vi "CRYDataView Pane Resize Proc.vi"(8 "DataView Index":i32, 11 "VI Ref":refnum<vi>) -> ()   [LabVIEW 2013]
uses:
  CRYNew View Global.vi
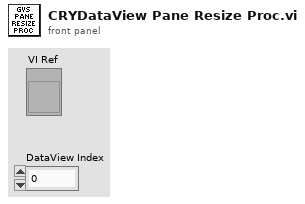
[diagram p1: front panel]
types:
  T1 = typedef "Graph Main Info Cluster.ctl" = cluster{"Selected_BarIdx":i32, "Selected_PanelIdx":i32, "Graph Main VIRef":refnum<vi>, "ToolBarClick":bool, "Spliter Ref Array":refnum<vi>[], "Panel Ref Array":refnum<vi>[], "Spliter_matrix":i32[][], "Panel_matrix":i32[][], "child_spliterIdx_matrix":i32[][], "split_pos_matrix":i32[][], "Title State":bool, "sQueueName":string, "Frame nID":i32, "Graph VIRef Array":cluster{"Graph VIRef":refnum<vi>, "Panel Idx":i32, "Frame VIRef":refnum<vi>, "Icon Ring":i32, "Graph Type":string}[], "View Type":string}
  T2 = typedef "LVRectTypeDef.ctl" = cluster{"Left":i16, "Top":i16, "Right":i16, "Bottom":i16}
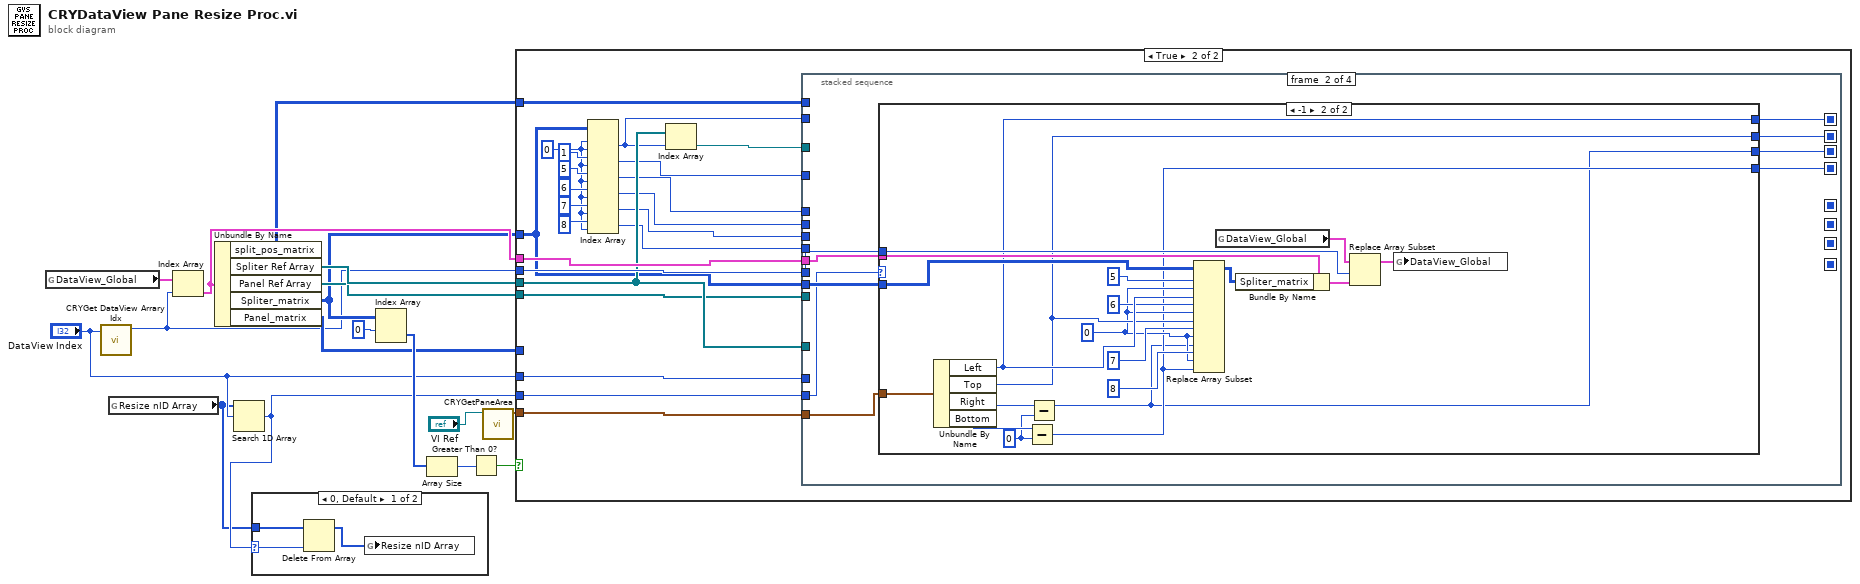
[diagram p0: block diagram]
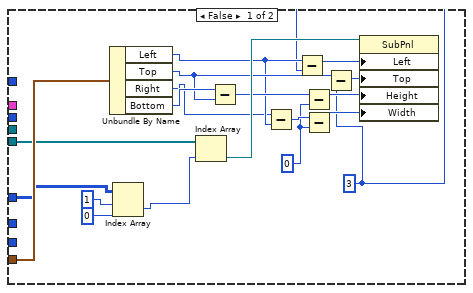
[diagram p3: hidden frame]
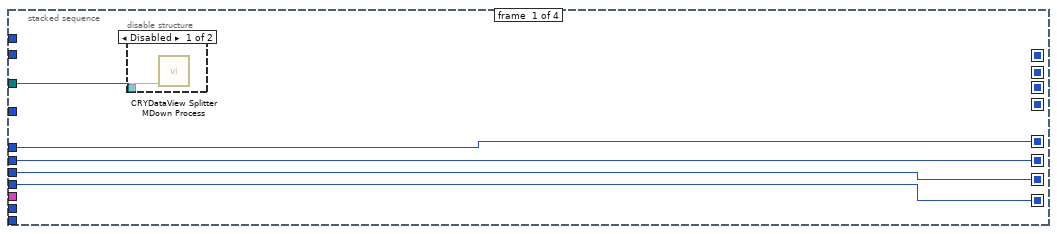
[diagram p4: hidden frame]
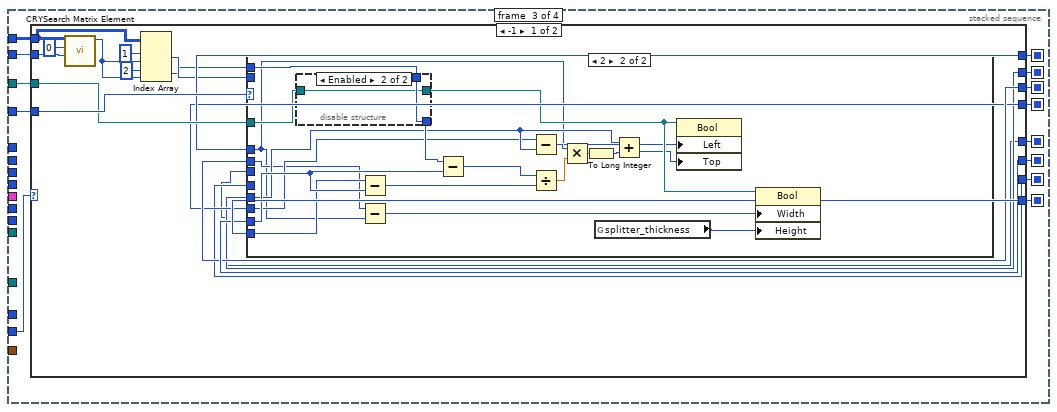
[diagram p7: hidden frame]
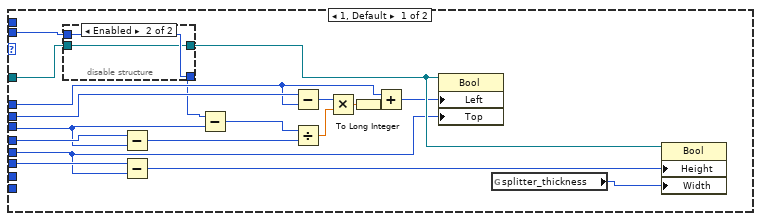
[diagram p8: hidden frame]
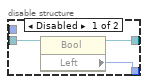
[diagram p9: hidden frame]
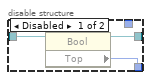
[diagram p10: hidden frame]
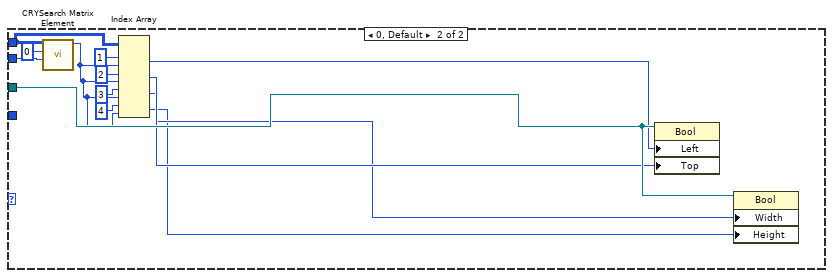
[diagram p11: hidden frame]
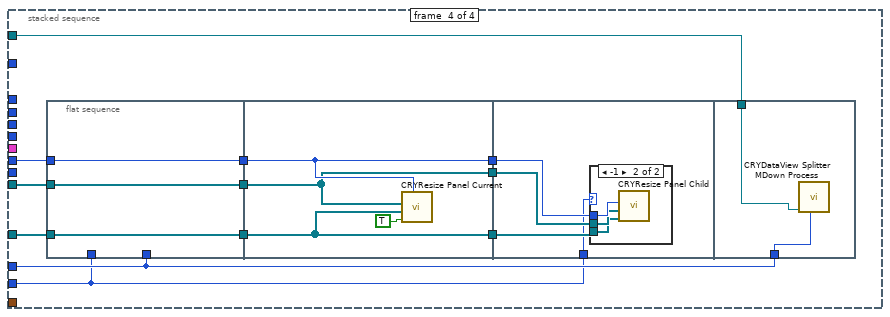
[diagram p12: hidden frame]
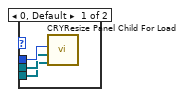
[diagram p13: hidden frame]
diagram:
  n1 = global read "CRYNew View Global.vi" "DataView_Global"() -> (w12:T1[])
  n2 = call "CRYGet DataView Arrary Idx.vi"("DataView Idx In"="DataView Index") -> ("DataView Arrary Idx out"=w5:i32)  [unwired: 10 in]
  n3 = global read "CRYNew View Global.vi" "Resize nID Array"() -> (w1:i32[])
  n4 = Index Array(array=w12, index=w5) -> (element=w13:T1)
  n5 = Unbundle By Name(w13) -> ("split_pos_matrix"=w4:i32[][], "Spliter Ref Array"=w10:refnum<vi>[], "Panel Ref Array"=w9:refnum<vi>[], "Spliter_matrix"=w6:i32[][], "Panel_matrix"=w7:i32[][])
  n6 = Search 1D Array(1D array=w1, element="DataView Index") -> (index of element=w2:i32)  [unwired: 1 in]
  n7 = case shown="0, Default" w2 {
    selector: w2 -> [w19 _]
    tunnel: w1 -> [w20 _]
    frame 0, Default {
      n8 = Delete From Array(array=w20, index=w19) -> (array with subset deleted=w18:i32[])  [unwired: 1 in, 1 out]
      n9 = global write "CRYNew View Global.vi" "Resize nID Array"(w18) -> ()
    }
    frame -1 {
    }
  }
  n10 = Index Array(array=w6, index (row)=0) -> (element=w16:i32[])  [unwired: 1 in]
  n11 = Array Size(array=w16) -> (size(s)=w15:i32)
  n12 = Greater Than 0?(x=w15) -> (x > 0?=w14:bool)
  n13 = call "CRYGetPaneArea.vi"("vi reference"="VI Ref") -> ("Content Area Rect"=w11:T2)  [unwired: 10 in]
  n14 = case shown="True" w14 {
    tunnel: w6 -> [_ w49]
    tunnel: w10 -> [_ w58]
    tunnel: w13 -> [_ w60]
    tunnel: w5 -> [_ w59]
    tunnel: w9 -> [w38 w57]
    tunnel: w11 -> [w39 w56]
    tunnel: w7 -> [w30 _]
    tunnel: "DataView Index" -> [_ w45]
    tunnel: w4 -> [_ w42]
    tunnel: w2 -> [_ w40]
    frame False {
      w21 = 3
      w24 = i16 0 ("y")
      n15 = Unbundle By Name(w39) -> ("Left"=w32:i16, "Top"=w35:i16, "Right"=w31:i16, "Bottom"=w36:i16)
      n16 = Index Array(array=w30, index (row)=1, index (col)=0) -> (element=w27:i32)
      n17 = Index Array(array=w38, index=w27) -> (element=w37:refnum<vi>)
      n18 = Subtract(x=w36, y=w35) -> (x-y=w34:i16)
      n19 = Subtract(x=w31, y=w32) -> (x-y=w33:i16)
      n20 = Subtract(x=w32, y=w21) -> (x-y=w23:i32)
      n21 = Subtract(x=w34, y=w24) -> (x-y=w25:i16)
      n22 = Subtract(x=w33, y=w24) -> (x-y=w26:i16)
      n23 = Subtract(x=w35, y=w21) -> (x-y=w22:i32)
      n24 = property class="SubPnl"(reference=w37, "Left"=w23, "Top"=w22, "Height"=w25, "Width"=w26) -> ()  [unwired: 1 in, 2 out]
    }
    frame True {
      w50 = 0 ("disabled index (col)")
      n25 = Index Array(array=w49, index (row) #1=w50, index (col) #1=w50, index (row) #2=1 ("index (row)"), index (col) #2=w50, index (row) #3=5 ("index (row)"), index (col) #3=w50, index (row) #4=6 ("index (row)"), index (col) #4=w50, index (row) #5=7 ("index (row)"), index (col) #5=w50, index (row) #6=8 ("index (row)"), index (col) #6=w50) -> (element #1=w41:i32, element #2=w48:i32, element #3=w47:i32, element #4=w46:i32, element #5=w44:i32, element #6=w43:i32)
      n26 = Index Array(array=w58, index=w41) -> (element=w61:refnum<vi>)
      n27 = stacked-sequence {
        seq-local: [w63 _ _ _] -> [_ _ w107 _]
        seq-local: [w64 _ _ _] -> [_ _ w101 _]
        seq-local: [w65 _ _ _] -> [_ _ w106 _]
        seq-local: [w66 _ _ _] -> [_ _ w100 _]
        seq-local: [_ w72 _ _] -> [_ _ w104 _]
        seq-local: [_ w71 _ _] -> [_ _ w102 _]
        seq-local: [_ w69 _ _] -> [_ _ w105 _]
        seq-local: [_ w70 _ _] -> [_ _ w103 _]
        tunnel: w61 -> [w62 _ w108 w194]
        tunnel: w60 -> [_ w76 _ _]
        tunnel: w49 -> [_ w73 _ _]
        tunnel: w59 -> [_ w75 _ w195]
        tunnel: w48 -> [_ _ w109 _]
        tunnel: w47 -> [w66 _ _ _]
        tunnel: w46 -> [w65 _ _ _]
        tunnel: w44 -> [w64 _ _ _]
        tunnel: w43 -> [w63 _ _ _]
        tunnel: w58 -> [_ _ _ w197]
        tunnel: w57 -> [_ _ _ w196]
        tunnel: w56 -> [_ w74 _ _]
        tunnel: w45 -> [_ _ _ w190]
        tunnel: w42 -> [_ _ w98 _]
        tunnel: w41 -> [_ _ w99 _]
        tunnel: w40 -> [_ w68 w97 w189]
        frame #0 {
          n28 = disable-structure shown="Disabled" {
            disable-tunnel: w62 -> [w67 _]
            frame Disabled {
              n29 = call "CRYDataView Splitter MDown Process.vi"("Selected Spliter Ref"=w67) -> ()  [unwired: 10 in, 1 out]
            }
            frame Enabled {
            }
          }
        }
        frame #1 {
          n30 = case shown="-1" w68 {
            tunnel: w76 -> [_ w96]
            tunnel: w75 -> [_ w94]
            tunnel: w74 -> [_ w91]
            tunnel: w73 -> [_ w90]
            tunnel: [_ w88] -> w72
            tunnel: [_ w86] -> w71
            tunnel: [_ w80] -> w70
            tunnel: [_ w78] -> w69
            frame 0, Default {
            }
            frame -1 {
              w77 = i16 0 ("y")
              w82 = 0 ("index (col)")
              n31 = Unbundle By Name(w91) -> ("Left"=w88:i16, "Top"=w86:i16, "Right"=w84:i16, "Bottom"=w79:i16)
              n32 = Subtract(x=w79, y=w77) -> (x-y=w80:i16)
              n33 = Subtract(x=w84, y=w77) -> (x-y=w78:i16)
              n34 = Replace Array Subset(array=w90, new element #1=w88, index (row) #1=5 ("disabled index (row)"), index (col) #1=w82, new element #2=w86, index (row) #2=6 ("disabled index (row)"), index (col) #2=w82, new element #3=w78, index (row) #3=7 ("disabled index (row)"), index (col) #3=w82, new element #4=w80, index (row) #4=8 ("disabled index (row)"), index (col) #4=w82) -> (w81:i32[][])
              n35 = global read "CRYNew View Global.vi" "DataView_Global"() -> (w92:T1[])
              n36 = Bundle By Name(cluster=w96, "Spliter_matrix"=w81) -> (w95:T1)
              n37 = Replace Array Subset(array=w92, new element=w95, index=w94) -> (w93:T1[])
              n38 = global write "CRYNew View Global.vi" "DataView_Global"(w93) -> ()
            }
          }
        }
        frame #2 {
          n39 = case shown="-1" w97 {
            tunnel: w109 -> [w127 _]
            tunnel: w108 -> [w126 w183]
            tunnel: w107 -> [w125 _]
            tunnel: w106 -> [w124 _]
            tunnel: w105 -> [w123 _]
            tunnel: w104 -> [w122 _]
            tunnel: w103 -> [w121 _]
            tunnel: w102 -> [w120 _]
            tunnel: w101 -> [w119 _]
            tunnel: w100 -> [w118 _]
            tunnel: w99 -> [w117 w188]
            tunnel: w98 -> [w115 w186]
            frame -1 {
              n40 = call "CRYSearch Matrix Element.vi"("element"=w117, "index (row)"=0, "matrix in"=w115) -> ("index of element"=w112:i32)  [unwired: 8 in]
              n41 = Index Array(array=w115, index (row) #1=1 ("disabled index (row)"), index (col) #1=w112, index (row) #2=2 ("disabled index (row)"), index (col) #2=w112) -> (element #1=w113:i32, element #2=w110:i32)
              n42 = case shown="2" w127 {
                tunnel: w126 -> [w136 w164]
                tunnel: w119 -> [w146 _]
                tunnel: w125 -> [_ w160]
                tunnel: w124 -> [_ w163]
                tunnel: w123 -> [w140 w159]
                tunnel: w122 -> [w139 w155]
                tunnel: w121 -> [w138 w161]
                tunnel: w120 -> [w130 w162]
                tunnel: w118 -> [w135 _]
                tunnel: w113 -> [w134 _]
                tunnel: w110 -> [_ w158]
                frame 1, Default {
                  n43 = disable-structure shown="Enabled" {
                    disable-tunnel: [w149 w151] -> w137
                    disable-tunnel: w136 -> [w148 w150]
                    disable-tunnel: [w147 w150] -> w133
                    disable-tunnel: w134 -> [_ w151]
                    frame Disabled {
                      n44 = property class="Bool"(reference=w148) -> (reference out=w147:refnum<vi>, "Left"=w149:i32)  [unwired: 1 in, 1 out]
                    }
                    frame Enabled {
                    }
                  }
                  n45 = Subtract(x=w146, y=w135) -> (x-y=w145:i32)
                  n46 = Subtract(x=w138, y=w130) -> (x-y=w129:i16)
                  n47 = Subtract(x=w137, y=w135) -> (x-y=w144:i32)
                  n48 = Subtract(x=w140, y=w139) -> (x-y=w141:i16)
                  n49 = Divide(x=w144, y=w145) -> (x/y=w143:dbl)
                  n50 = Multiply(x=w141, y=w143) -> (x*y=w142:dbl)
                  n51 = To Long Integer(number=w142) -> (32bit integer=w132:i32)
                  n52 = Add(x=w139, y=w132) -> (x+y=w131:i32)
                  n53 = property class="Bool"(reference=w133, "Left"=w131, "Top"=w130) -> ()  [unwired: 1 in, 2 out]
                  n54 = global read "CRYNew View Global.vi" "splitter_thickness"() -> (w128:u32)
                  n55 = property class="Bool"(reference=w133, "Height"=w129, "Width"=w128) -> ()  [unwired: 1 in, 2 out]
                }
                frame 2 {
                  n56 = disable-structure shown="Enabled" {
                    disable-tunnel: [w173 w175] -> w165
                    disable-tunnel: w164 -> [w172 w174]
                    disable-tunnel: [w171 w174] -> w156
                    disable-tunnel: w158 -> [_ w175]
                    frame Disabled {
                      n57 = property class="Bool"(reference=w172) -> (reference out=w171:refnum<vi>, "Top"=w173:i32)  [unwired: 1 in, 1 out]
                    }
                    frame Enabled {
                    }
                  }
                  n58 = Subtract(x=w160, y=w163) -> (x-y=w170:i32)
                  n59 = Subtract(x=w159, y=w155) -> (x-y=w153:i16)
                  n60 = Subtract(x=w165, y=w163) -> (x-y=w169:i32)
                  n61 = Subtract(x=w161, y=w162) -> (x-y=w166:i16)
                  n62 = Divide(x=w169, y=w170) -> (x/y=w168:dbl)
                  n63 = Multiply(x=w166, y=w168) -> (x*y=w167:dbl)
                  n64 = To Long Integer(number=w167) -> (32bit integer=w157:i32)
                  n65 = global read "CRYNew View Global.vi" "splitter_thickness"() -> (w152:u32)
                  n66 = Add(x=w162, y=w157) -> (x+y=w154:i32)
                  n67 = property class="Bool"(reference=w156, "Left"=w155, "Top"=w154) -> ()  [unwired: 1 in, 2 out]
                  n68 = property class="Bool"(reference=w156, "Width"=w153, "Height"=w152) -> ()  [unwired: 1 in, 2 out]
                }
              }
            }
            frame 0, Default {
              n69 = call "CRYSearch Matrix Element.vi"("element"=w188, "index (row)"=0, "matrix in"=w186) -> ("index of element"=w180:i32)  [unwired: 8 in]
              n70 = Index Array(array=w186, index (row) #1=1 ("disabled index (row)"), index (col) #1=w180, index (row) #2=2 ("disabled index (row)"), index (col) #2=w180, index (row) #3=3 ("disabled index (row)"), index (col) #3=w180, index (row) #4=4 ("disabled index (row)"), index (col) #4=w180) -> (element #1=w179:i32, element #2=w178:i32, element #3=w177:i32, element #4=w176:i32)
              n71 = property class="Bool"(reference=w183, "Left"=w179, "Top"=w178) -> ()  [unwired: 1 in, 2 out]
              n72 = property class="Bool"(reference=w183, "Width"=w177, "Height"=w176) -> ()  [unwired: 1 in, 2 out]
            }
          }
        }
        frame #3 {
          n73 = flat-sequence {
            tunnel: w195 -> [w202]
            tunnel: w197 -> [w201]
            tunnel: w196 -> [w203]
            tunnel: [w203] -> w193
            tunnel: [w201] -> w192
            tunnel: [w202] -> w191
            tunnel: w190 -> [_]
            tunnel: w189 -> [_]
            tunnel: [w206] -> w200
            tunnel: [w205] -> w199
            tunnel: [w204] -> w198
            tunnel: w193 -> [w205]
            tunnel: w192 -> [w204]
            tunnel: w191 -> [w206]
            tunnel: w200 -> [w211]
            tunnel: w199 -> [w210]
            tunnel: w198 -> [w209]
            tunnel: w189 -> [w208]
            tunnel: w194 -> [w219]
            tunnel: w190 -> [w218]
            frame #0 {
            }
            frame #1 {
              n74 = call "CRYResize Panel Current.vi"("DataView Array Idx"=w206, "close_panel"=TRUE, "spliter array"=w204, "SubPanel array"=w205) -> ()  [unwired: 8 in]
            }
            frame #2 {
              n75 = case shown="-1" w208 {
                tunnel: w211 -> [w214 w217]
                tunnel: w210 -> [w213 w216]
                tunnel: w209 -> [w212 w215]
                frame 0, Default {
                  n76 = call "CRYResize Panel Child For Load.vi"("spliter array"=w212, "SubPanel array"=w213, "DataView Array Idx"=w214) -> ()  [unwired: 9 in]
                }
                frame -1 {
                  n77 = call "CRYResize Panel Child.vi"("spliter array"=w215, "SubPanel array"=w216, "DataView Array Idx"=w217) -> ()  [unwired: 9 in]
                }
              }
            }
            frame #3 {
              n78 = call "CRYDataView Splitter MDown Process.vi"("DataView Index"=w218, "Selected Spliter Ref"=w219) -> ()  [unwired: 9 in, 1 out]
            }
          }
        }
      }
    }
  }
